vi "Autosampler Set Fill Volume.vi"(7 "Correlation ID":u32, 8 "error in (no error)":errorcluster, 10 "Volume, uL":u16, 11 "Application in":refnum<class "Application.lvclass">) -> (0 "error out":errorcluster, 3 "Application out":refnum<class "Application.lvclass">)   [LabVIEW 2023, in "Application.lvlib" / "Application.lvclass"]
uses:
  Application.lvclass
  Application.lvclass/Application.ctl
  Hardware/Device Messages/Save CorrID Msg/Save CorrID Msg.lvclass
  Hardware/Autosampler Messages/Set Fill Volume Msg/Set Fill Volume Msg.lvclass
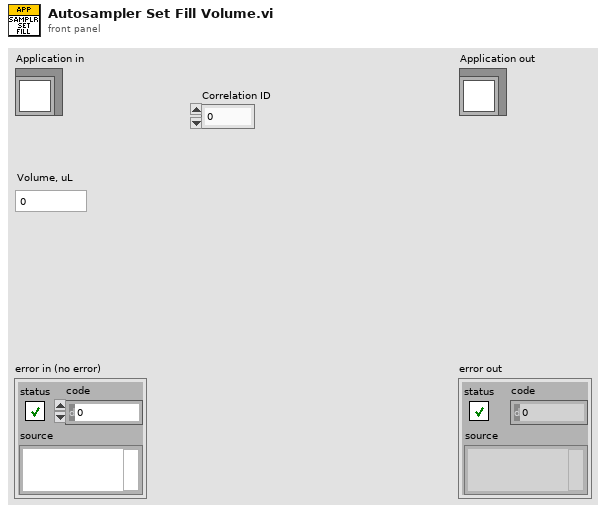
[diagram p1: front panel]
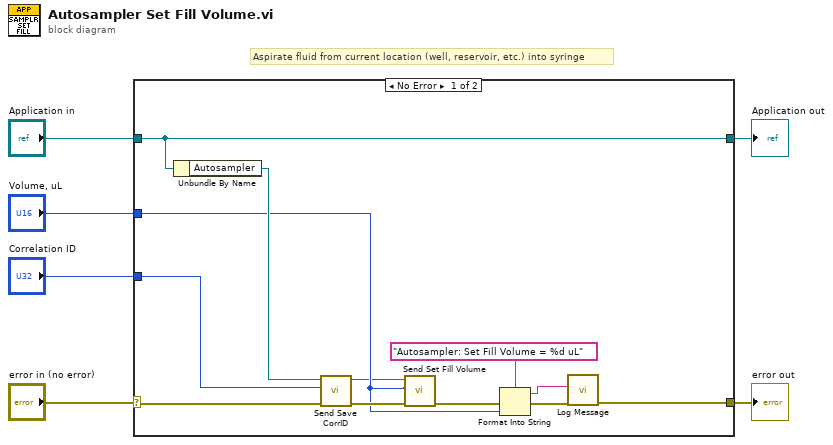
[diagram p0: block diagram]
diagram:
  # "Aspirate fluid from current location (well, reservoir, etc.) into syringe"
  n1 = case shown="No Error" "error in (no error)" {
    selector: "error in (no error)" -> [w12 w20]
    tunnel: [w17 w20] -> w5
    tunnel: [w18 w19] -> w3
    tunnel: "Application in" -> [w18 w19]
    tunnel: "Volume, uL" -> [w9 _]
    tunnel: "Correlation ID" -> [w11 _]
    frame No Error {
      n2 = Unbundle By Name(w18) -> ("Autosampler"=w13:refnum<class "Message Enqueuer.lvclass">)
      n3 = call "Send Save CorrID.vi"("error in (no error)"=w12, "Correlation ID"=w11, "Message Enqueuer"=w13) -> ("error out"=w10:errorcluster, "Message Enqueuer out"=w8:refnum<class "Message Enqueuer.lvclass">)  [unwired: 7 in]
      n4 = call "Send Set Fill Volume.vi"("error in (no error)"=w10, "Volume, uL"=w9, "Message Enqueuer"=w8) -> ("error out"=w7:errorcluster)  [unwired: 7 in, 1 out]
      n5 = Format Into String(format string="Autosampler: Set Fill Volume = %d uL", error in=w7, w9) -> (resulting string=w16:string, error out=w15:errorcluster)  [unwired: 1 in]
      n6 = call "Log Message.vi"("error constant"=w15, "input"=w16) -> ("error constant 2"=w17:errorcluster)  [unwired: 8 in, 1 out]
    }
    frame Error {
    }
  }
  "error out" <- w5
  "Application out" <- w3
